vi "WS_RS485ETH_command.vi"(5 "action":enum16{"Request", "Control"}(ring), 6 "do_read":bool=TRUE, 7 "device_addr":u16=22, 8 "error in":errorcluster, 9 "data_string":string="1", 10 "param_num":u16=22, 11 "conn_id_in":refnum<k5>) -> (0 "error out":errorcluster, 1 "data_out":string, 2 "response":string, 3 "conn_id_out":refnum<k5>, 4 "status":bool)   [LabVIEW 2019]
panel:
  in  "timeout ms":i32=1000
  out "command":string
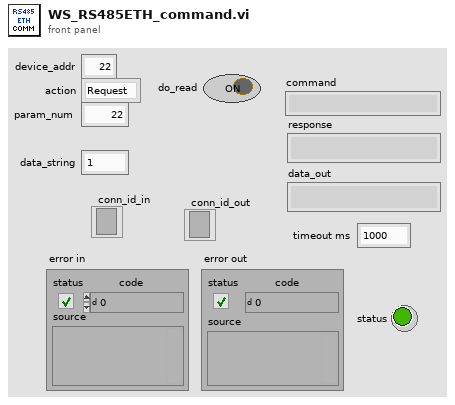
[diagram p1: front panel]
types:
  T1 = enum16{"Standard", "Buffered", "CRLF", "Immediate"}
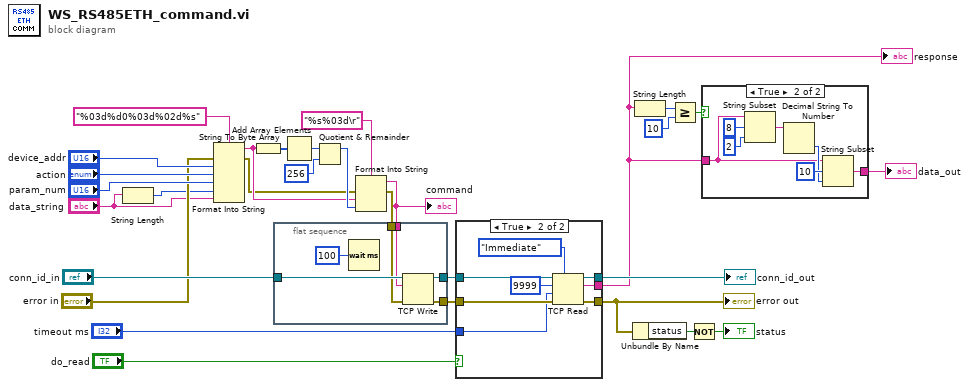
[diagram p0: block diagram]
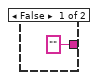
[diagram p2: hidden frame]
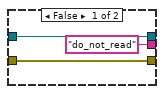
[diagram p3: hidden frame]
diagram:
  n1 = String Length(string="data_string") -> (length=w7:i32)
  n2 = Format Into String(format string="%03d%d0%03d%02d%s", error in="error in", "device_addr", "action", "param_num", w7, "data_string") -> (resulting string=w11:string, error out=w9:errorcluster)  [unwired: 1 in]
  n3 = String To Byte Array(string=w11) -> (unsigned byte array=w23:u8[])
  n4 = flat-sequence {
    tunnel: [w36] -> w30
    tunnel: [w35] -> w29
    tunnel: "conn_id_in" -> [w34]
    tunnel: w19 -> [w33]
    tunnel: w18 -> [w32]
    frame #0 {
      n5 = Wait (ms)(milliseconds to wait=u32 100) -> ()  [unwired: 1 out]
      n6 = TCP Write(connection ID=w34, data in=w33, error in (no error)=w32) -> (connection ID out=w35:refnum<k5>, error out=w36:errorcluster)  [unwired: 1 in, 1 out]
    }
  }
  n7 = Add Array Elements(numeric array=w23) -> (sum=w21:u8)
  n8 = Quotient & Remainder(x=w21, y=u64 256) -> (x-y*floor(x/y)=w16:u64)  [unwired: 1 out]
  n9 = Format Into String(format string="%s%03d\r", error in=w9, w11, w16) -> (resulting string=w19:string, error out=w18:errorcluster)  [unwired: 1 in]
  "command" <- w19
  n10 = case shown="True" "do_read" {
    tunnel: w30 -> [w38 w47]
    tunnel: w29 -> [w39 w46]
    tunnel: [w39 w43] -> w28
    tunnel: [w38 w42] -> w26
    tunnel: ["do_not_read" ("data out") w41] -> w2
    tunnel: "timeout ms" -> [_ w40]
    frame False {
    }
    frame True {
      n11 = TCP Read(connection ID=w46, bytes to read=9999, error in (no error)=w47, 7:T1."Immediate" ("mode (standard)"), 9:w40) -> (connection ID out=w43:refnum<k5>, data out=w41:string, error out=w42:errorcluster)
    }
  }
  "error out" <- w26
  "response" <- w2
  "conn_id_out" <- w28
  n12 = Unbundle By Name(w26) -> ("status"=w25:bool)
  n13 = String Length(string=w2) -> (length=w5:i32)
  n14 = Greater Or Equal?(x=w5, y=10) -> (x >= y?=w3:bool)
  n15 = Not(x=w25) -> (.not. x?=→"status":bool)
  n16 = case shown="True" w3 {
    tunnel: w2 -> [_ w50]
    tunnel: ["" ("data out") w49] -> w1
    frame False {
    }
    frame True {
      n17 = String Subset(string=w50, offset (0)=8, length (rest)=2 ("length (rest)")) -> (substring=w52:string)
      n18 = Decimal String To Number(string=w52) -> (number=w51:i32)  [unwired: 2 in, 1 out]
      n19 = String Subset(string=w50, offset (0)=10, length (rest)=w51) -> (substring=w49:string)
    }
  }
  "data_out" <- w1
